vi "Config.vi"(7 "delay (5ms)":u32=5, 8 "error in (no error)":errorcluster, 11 "PORT (GPIB)":refnum<visa-resource-name>) -> (0 "error out":errorcluster, 3 "Reference out":T1={"Device"="", "Function"="", "delay"=20, "Resolution"=0})   [LabVIEW 2021, in "Rigol DM3052.lvlib"]
uses:
  Rigol DM3052.lvlib
  Reference.ctl
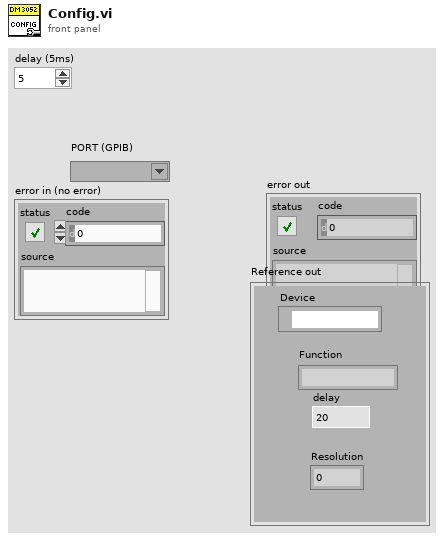
[diagram p1: front panel]
types:
  T1 = typedef "Rigol DM3052.lvlib/Reference.ctl" = cluster{"Device":refnum<visa-resource-name>, "Function":string, "delay":u32, "Resolution":i8}
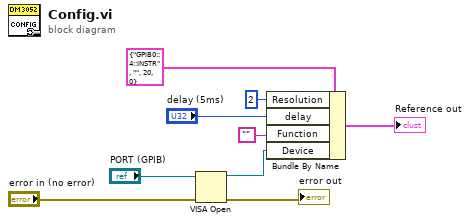
[diagram p0: block diagram]
diagram:
  n1 = VISA Open(error in (no error)="error in (no error)", VISA resource name="PORT (GPIB)") -> (VISA resource name=w5:refnum<visa-resource-name>, error out=→"error out":errorcluster)  [unwired: 3 in]
  n2 = Bundle By Name(cluster=T1 {"Device"="GPIB0::4::INSTR", "Function"="", "delay"=20, "Resolution"=0} ("Reference out"), "Resolution"=i8 2, "delay"="delay (5ms)", "Function"="", "Device"=w5) -> (→"Reference out":T1)
